vi "enumerateStaticDependencies.vi"(8 "error in (no error)":errorcluster, 11 "Instrument.DAQ":refnum<class "Instrument.DAQ.lvclass">) -> (0 "error out":errorcluster, 2 "Static Dependencies":refnum<class "Dependency.lvclass">[](array[class]), 3 "Instrument.DAQ out":refnum<class "Instrument.DAQ.lvclass">)   [LabVIEW 2019, in "Instrument.Lockin.lvlib" / "Instrument.DAQ.lvclass"]
uses:
  Instrument.DAQ.lvclass
  <vilib>/JKI/JKI SMO/Dependency/Dependency.lvclass
  Instrument.DAQ.lvclass/Instrument.DAQ.ctl
  Generator/Generator.lvclass/Generator.ctl
  DAQmx/DAQmx.lvclass
  C:/Program Files/National Instruments/LabVIEW 2019/vi.lib/JKI/JKI SMO/SMO/SMO.lvclass
  Generator/Generator.lvclass
  <vilib>/JKI/JKI SMO/SMO/SMO.lvclass
panel:
  # "For instructions on how to use the JKI State Machine Objects, examples and video tutorials, visit:\nhttp://jki.net/state-machine-objects/\n\nJKI State Machine Objects™\nhttp://jki.net/state-machine-objects/\nCopyright (C) 2005-2015, JKI <info@jki.net>\nALL RIGHTS RESERVED"
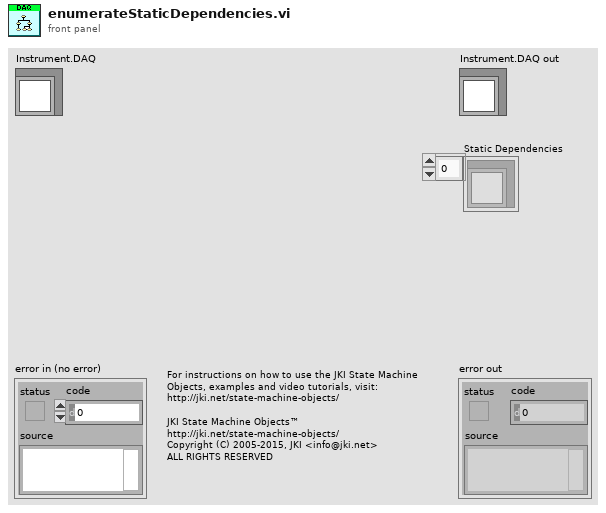
[diagram p1: front panel]
types:
  T1 = typedef "DAQmx.lvclass/PublicQueues--Cluster.ctl" = cluster{"AO":refnum<queue>, "REF_X":refnum<queue>, "REF_Y":refnum<queue>}
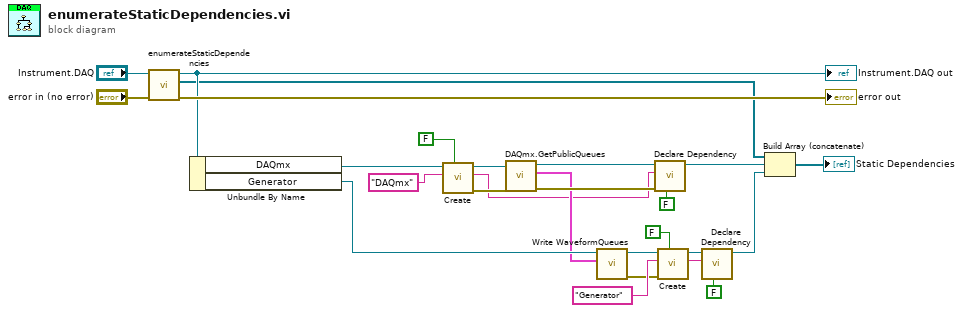
[diagram p0: block diagram]
diagram:
  n1 = call-parent "enumerateStaticDependencies.vi"("error in (no error)"="error in (no error)", "SMO"="Instrument.DAQ") -> ("error out"=→"error out":errorcluster, "Static Dependencies"=w13:refnum<class "Dependency.lvclass">[], "SMO out"=w21:refnum<class "Instrument.DAQ.lvclass">)  [unwired: 7 in]
  "Instrument.DAQ out" <- w21
  n2 = Unbundle By Name(w21) -> ("DAQmx"=w6:refnum<class "DAQmx.lvclass">, "Generator"=w10:refnum<class "Generator.lvclass">)
  n3 = call <vilib>:"Create.vi"("Shared Resource (F)"=FALSE, "Subsystem Name (optional)"="DAQmx" ("Name"), "SMO"=w6) -> ("error out"=w4:errorcluster, "SMO name"=w3:string, "SMO out"=w5:refnum<class "DAQmx.lvclass">)  [unwired: 6 in]
  n4 = call "DAQmx.GetPublicQueues.vi"("error in (no error)"=w4, "DAQmx"=w5) -> ("error out"=w11:errorcluster, "Public Queues"=w9:T1, "DAQmx out"=w12:refnum<class "DAQmx.lvclass">)  [unwired: 7 in]
  n5 = call "Write WaveformQueues.vi"("WaveformQueues"=w9, "Generator in"=w10) -> ("error out"=w7:errorcluster, "Generator out"=w8:refnum<class "Generator.lvclass">)  [unwired: 8 in]
  n6 = call <vilib>:"Declare Dependency.vi"("Shared Resource (F)"=FALSE, "error in (no error)"=w11, "Name"=w3, "Type"=w12) -> ("Dependency out"=w22:refnum<class "Dependency.lvclass">)  [unwired: 6 in, 1 out]
  n7 = call <vilib>:"Create.vi"("Shared Resource (F)"=FALSE, "error in (no error)"=w7, "Subsystem Name (optional)"="Generator" ("Name"), "SMO"=w8) -> ("SMO name"=w15:string, "SMO out"=w16:refnum<class "Generator.lvclass">)  [unwired: 5 in, 1 out]
  n8 = call <vilib>:"Declare Dependency.vi"("Shared Resource (F)"=FALSE, "Name"=w15, "Type"=w16) -> ("Dependency out"=w18:refnum<class "Dependency.lvclass">)  [unwired: 7 in, 1 out]
  n9 = Build Array (concatenate)(w13, w22, w18) -> (→"Static Dependencies":refnum<class "Dependency.lvclass">[])
